vi "Palette mockup.vi"   [LabVIEW 2017, in "Switch Scripting.lvlib"]
uses:
  Switch Scripting.lvlib
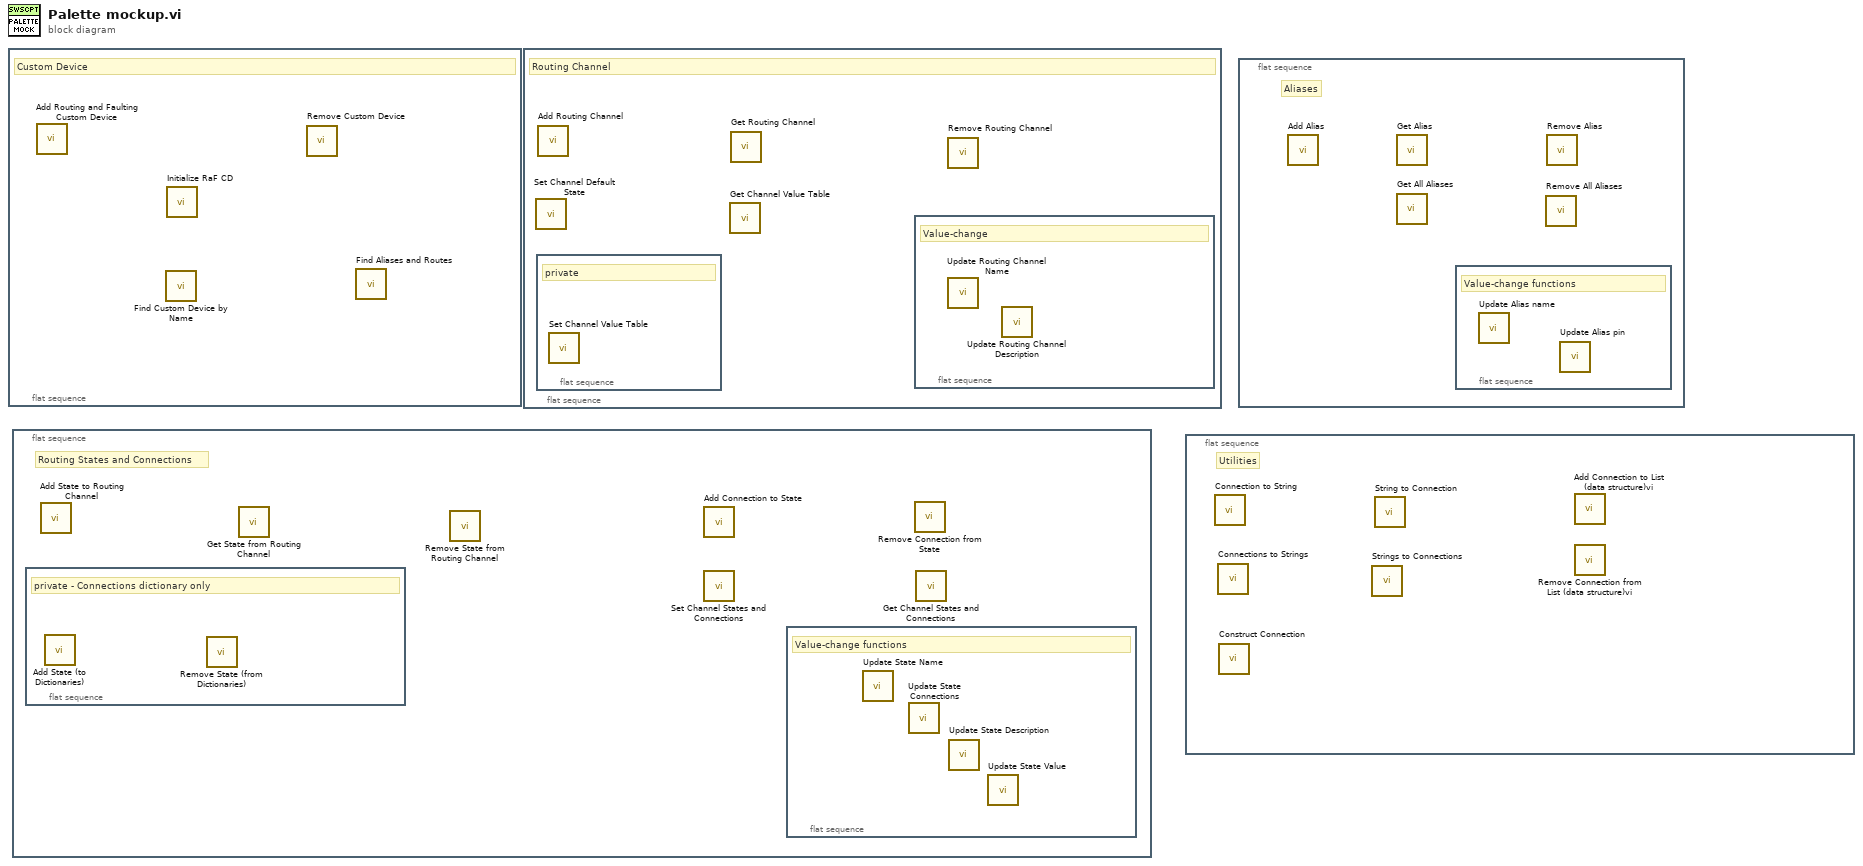
[diagram p0: block diagram]
diagram:
  n1 = flat-sequence {
    frame #0 {
      # "Custom Device"
      n2 = call "Add Routing and Faulting Custom Device.vi"() -> ()  [unwired: 11 in, 5 out]
      n3 = call "Find Custom Device by Name.vi"() -> ()  [unwired: 9 in, 3 out]
      n4 = call "Initialize RaF CD.vi"() -> ()  [unwired: 8 in, 4 out]
      n5 = call "Remove Custom Device.vi"() -> ()  [unwired: 11 in, 1 out]
      n6 = call "Find Aliases and Routes.vi"() -> ()  [unwired: 8 in, 4 out]
    }
  }
  n7 = flat-sequence {
    frame #0 {
      # "Routing States and Connections"
      n8 = flat-sequence {
        frame #0 {
          # "private - Connections dictionary only"
          n9 = call "Add State (to Dictionaries).vi"() -> ()  [unwired: 10 in, 2 out]
          n10 = call "Remove State (from Dictionaries).vi"() -> ()  [unwired: 10 in, 2 out]
        }
      }
      n11 = call "Add State to Routing Channel.vi"() -> ()  [unwired: 10 in, 2 out]
      n12 = call "Get State from Routing Channel.vi"() -> ()  [unwired: 9 in, 3 out]
      n13 = call "Remove State from Routing Channel.vi"() -> ()  [unwired: 10 in, 2 out]
      n14 = call "Add Connection to State.vi"() -> ()  [unwired: 10 in, 2 out]
      n15 = call "Set Channel States and Connections.vi"() -> ()  [unwired: 10 in, 2 out]
      n16 = flat-sequence {
        frame #0 {
          # "Value-change functions"
          n17 = call "Update State Name.vi"() -> ()  [unwired: 10 in, 2 out]
          n18 = call "Update State Connections.vi"() -> ()  [unwired: 10 in, 2 out]
          n19 = call "Update State Description.vi"() -> ()  [unwired: 10 in, 2 out]
          n20 = call "Update State Value.vi"() -> ()  [unwired: 10 in, 2 out]
        }
      }
      n21 = call "Remove Connection from State.vi"() -> ()  [unwired: 9 in, 3 out]
      n22 = call "Get Channel States and Connections.vi"() -> ()  [unwired: 9 in, 3 out]
    }
  }
  n23 = flat-sequence {
    frame #0 {
      # "Routing Channel"
      n24 = call "Set Channel Default State.vi"() -> ()  [unwired: 10 in, 2 out]
      n25 = flat-sequence {
        frame #0 {
          # "private"
          n26 = call "Set Channel Value Table.vi"() -> ()  [unwired: 10 in, 2 out]
        }
      }
      n27 = call "Add Routing Channel.vi"() -> ()  [unwired: 13 in, 3 out]
      n28 = call "Get Channel Value Table.vi"() -> ()  [unwired: 8 in, 4 out]
      n29 = call "Get Routing Channel.vi"() -> ()  [unwired: 11 in, 5 out]
      n30 = flat-sequence {
        frame #0 {
          # "Value-change"
          n31 = call "Update Routing Channel Name.vi"() -> ()  [unwired: 14 in, 2 out]
          n32 = call "Update Routing Channel Description.vi"() -> ()  [unwired: 14 in, 2 out]
        }
      }
      n33 = call "Remove Routing Channel.vi"() -> ()  [unwired: 10 in, 2 out]
    }
  }
  n34 = flat-sequence {
    frame #0 {
      # "Utilities"
      n35 = call "Connection to String.vi"() -> ()  [unwired: 11 in, 1 out]
      n36 = call "Connections to Strings.vi"() -> ()  [unwired: 11 in, 1 out]
      n37 = call "Construct Connection.vi"() -> ()  [unwired: 11 in, 1 out]
      n38 = call "Strings to Connections.vi"() -> ()  [unwired: 11 in, 1 out]
      n39 = call "String to Connection.vi"() -> ()  [unwired: 11 in, 1 out]
      n40 = call "Add Connection to List (data structure)vi.vi"() -> ()  [unwired: 9 in, 3 out]
      n41 = call "Remove Connection from List (data structure)vi.vi"() -> ()  [unwired: 9 in, 3 out]
    }
  }
  n42 = flat-sequence {
    frame #0 {
      # "Aliases"
      n43 = call "Add Alias.vi"() -> ()  [unwired: 10 in, 2 out]
      n44 = call "Get Alias.vi"() -> ()  [unwired: 8 in, 4 out]
      n45 = call "Get All Aliases.vi"() -> ()  [unwired: 8 in, 4 out]
      n46 = flat-sequence {
        frame #0 {
          # "Value-change functions"
          n47 = call "Update Alias name.vi"() -> ()  [unwired: 10 in, 2 out]
          n48 = call "Update Alias pin.vi"() -> ()  [unwired: 9 in, 3 out]
        }
      }
      n49 = call "Remove All Aliases.vi"() -> ()  [unwired: 9 in, 3 out]
      n50 = call "Remove Alias.vi"() -> ()  [unwired: 9 in, 3 out]
    }
  }
